vi "SRV_VIG_JPEGtoPict.vi"(6 "Method (Get)":enum16{"Get", "Set"}(ring)) -> (1 "Mac JPEG Temp Image Path":path, 3 "Windows labjpeg7 DLL Path":path)   [LabVIEW 2014]
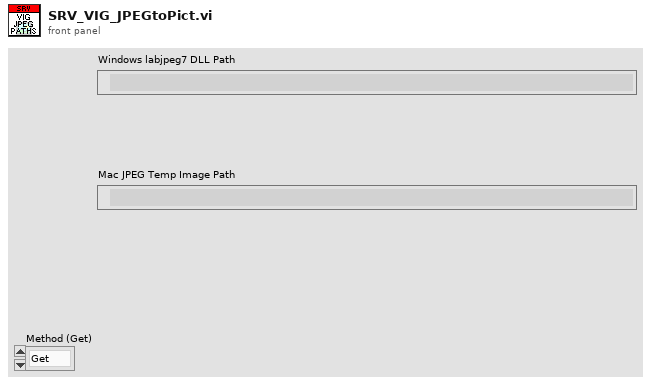
[diagram p1: front panel]
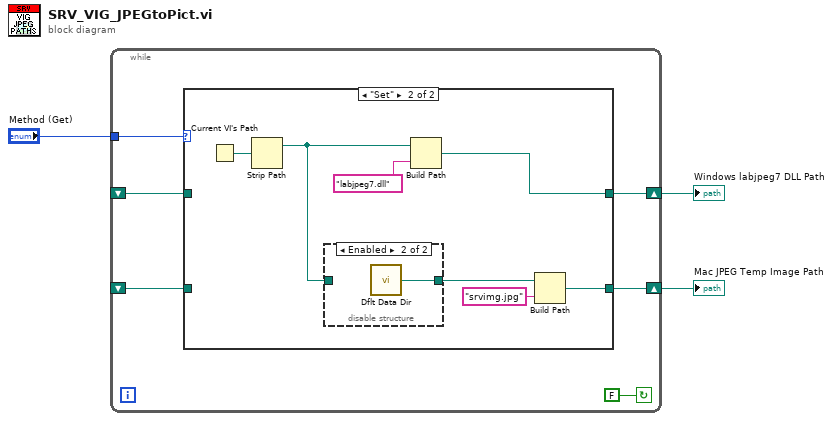
[diagram p0: block diagram]
diagram:
  n1 = while {
    tunnel: "Method (Get)" -> [w8]
    shift-right: [w5] -> w2
    shift-left: _ -> [w7]
    shift-right: [w4] -> w1
    shift-left: _ -> [w6]
    stop <- FALSE continue-if-true
    n2 = case shown="\"Set\"" w8 {
      tunnel: w7 -> [w11 _]
      tunnel: w6 -> [w10 _]
      tunnel: [w11 w16] -> w5
      tunnel: [w10 w14] -> w4
      frame "Get" {
      }
      frame "Set" {
        n3 = Current VI's Path() -> (path=w18:path)
        n4 = Strip Path(path=w18) -> (stripped path=w13:path)  [unwired: 1 out]
        n5 = disable-structure shown="Enabled" {
          disable-tunnel: w13 -> [w19 _]
          disable-tunnel: [w19 w20] -> w12
          frame Disabled {
          }
          frame Enabled {
            n6 = call <vilib>:"Dflt Data Dir.vi"() -> ("App:Default Data Directory"=w20:path)
          }
        }
        n7 = Build Path(base path=w13, name or relative path="labjpeg7.dll") -> (appended path=w16:path)
        n8 = Build Path(base path=w12, name or relative path="srvimg.jpg") -> (appended path=w14:path)
      }
    }
  }
  "Windows labjpeg7 DLL Path" <- w2
  "Mac JPEG Temp Image Path" <- w1
